vi "Lab Panel V5.31.vi"() -> ()   [LabVIEW 2017] (continued)
              tunnel: w5237 -> [w5242 _]
              tunnel: w5226 -> [_ w5275]
              tunnel: w5236 -> [_ w5274]
              tunnel: w5235 -> [_ w5273]
              tunnel: w5234 -> [_ w5272]
              tunnel: w5233 -> [_ w5271]
              tunnel: w5232 -> [_ w5270]
              tunnel: w5231 -> [_ w5269]
              tunnel: w5230 -> [_ w5268]
              tunnel: w5229 -> [_ w5267]
              tunnel: w5228 -> [_ w5266]
              tunnel: w5227 -> [_ w5265]
              tunnel: "TO (string):" -> [w5241 _]
              frame #0 {
                # "mail test"
                n2904 = case shown="True" w5242 {
                  tunnel: w5245 -> [_ w5249]
                  tunnel: w5241 -> [_ w5248]
                  tunnel: w5244 -> [_ w5247]
                  tunnel: w5243 -> [_ w5246]
                  frame False {
                  }
                  frame True {
                    n2905 = stacked-sequence {
                      seq-local: [_ _ w5259 _] -> [_ _ _ w5260]
                      tunnel: w5249 -> [w5252 _ _ w5264]
                      tunnel: w5248 -> [_ _ w5257 _]
                      tunnel: w5247 -> [_ _ w5255 _]
                      tunnel: w5246 -> [_ _ w5256 _]
                      frame #0 {
                        n2906 = Bundle(cluster=w5252, "TEST MAIL STATUS"="TEST START") -> (w5250:T8)  [unwired: 6 in]
                        n2907 = local write "MAIL SETTINGS"(w5250) -> ()
                      }
                      frame #1 {
                        n2908 = Wait (ms)(milliseconds to wait=500) -> ()  [unwired: 1 out]
                      }
                      frame #2 {
                        n2909 = call "sub vi - send mail v5.vi"("TO:"=w5257, "subject"="MAIL TEST FROM LAB PANEL", "from"=w5256, "out going server"=w5255, "message"="TEST MESSAGE") -> ("error out"=w5259:errorcluster)  [unwired: 10 in]
                      }
                      frame #3 {
                        n2910 = Bundle(cluster=w5264, "TEST MAIL"=FALSE, "TEST MAIL STATUS"="TEST END", "mail error"=w5260) -> (w5262:T8)  [unwired: 4 in]
                        n2911 = local write "MAIL SETTINGS"(w5262) -> ()
                      }
                    }
                  }
                }
              }
              frame #1 {
                # "mail report"
                n2912 = stacked-sequence {
                  seq-local: [_ w5322 _ _] -> [_ _ _ w5512]
                  seq-local: [_ _ w5425 _] -> [_ _ _ w5502]
                  seq-local: [w5289 _ _ _] -> [_ w5339 _ _]
                  seq-local: [w5288 _ _ _] -> [_ w5338 _ _]
                  seq-local: [w5286 _ _ _] -> [_ w5336 _ _]
                  seq-local: [w5287 _ _ _] -> [_ w5337 _ _]
                  seq-local: [w5285 _ _ _] -> [_ w5335 _ _]
                  seq-local: [w5284 _ _ _] -> [_ w5330 _ _]
                  seq-local: [w5283 _ _ _] -> [_ w5331 _ _]
                  seq-local: [w5282 _ _ _] -> [_ w5332 _ _]
                  seq-local: [w5281 _ _ _] -> [_ w5333 _ _]
                  seq-local: [w5280 _ _ _] -> [_ w5334 _ _]
                  tunnel: w5279 -> [_ _ _ w5513]
                  tunnel: w5278 -> [_ _ _ w5496]
                  tunnel: w5277 -> [_ _ _ w5510]
                  tunnel: w5276 -> [_ _ _ w5509]
                  tunnel: w5275 -> [w5320 _ _ w5504]
                  tunnel: w5274 -> [_ _ w5455 _]
                  tunnel: w5273 -> [_ _ w5452 _]
                  tunnel: w5272 -> [_ _ w5451 _]
                  tunnel: w5271 -> [_ _ w5450 _]
                  tunnel: w5270 -> [_ _ w5449 _]
                  tunnel: w5269 -> [_ _ w5448 _]
                  tunnel: w5268 -> [_ _ w5447 _]
                  tunnel: w5267 -> [_ _ w5446 _]
                  tunnel: w5266 -> [_ _ w5445 _]
                  tunnel: w5265 -> [_ _ w5444 _]
                  frame #0 {
                    n2913 = case shown="False" w5320 {
                      frame False {
                        n2914 = local write "mail control"("") -> ()
                      }
                      frame True {
                      }
                    }
                    n2915 = local read "SET LAB01-1"() -> (w5319:T6)
                    n2916 = local read "SET LAB01-2"() -> (w5318:T5)
                    n2917 = local read "SET LAB02-1"() -> (w5317:T5)
                    n2918 = local read "SET LAB02-2"() -> (w5316:T5)
                    n2919 = local read "SET LAB03-1"() -> (w5315:T5)
                    n2920 = local read "SET LAB04-1"() -> (w5313:T5)
                    n2921 = local read "SET LAB05-1"() -> (w5311:T5)
                    n2922 = local read "SET LAB03-2"() -> (w5314:T5)
                    n2923 = local read "SET LAB04-2"() -> (w5312:T5)
                    n2924 = local read "SET LAB05-2"() -> (w5310:T5)
                    n2925 = Unbundle(w5315) -> ("DESCRIPTION"=w5295:string)  [unwired: 4 out]
                    n2926 = Unbundle(w5314) -> ("DESCRIPTION"=w5294:string)  [unwired: 4 out]
                    n2927 = Unbundle(w5313) -> ("DESCRIPTION"=w5293:string)  [unwired: 4 out]
                    n2928 = Unbundle(w5310) -> ("DESCRIPTION"=w5290:string)  [unwired: 4 out]
                    n2929 = Unbundle(w5316) -> ("DESCRIPTION"=w5296:string)  [unwired: 4 out]
                    n2930 = Unbundle(w5312) -> ("DESCRIPTION"=w5292:string)  [unwired: 4 out]
                    n2931 = Unbundle(w5319) -> ("DESCRIPTION"=w5308:string)  [unwired: 4 out]
                    n2932 = Unbundle(w5317) -> ("DESCRIPTION"=w5297:string)  [unwired: 4 out]
                    n2933 = Unbundle(w5311) -> ("DESCRIPTION"=w5291:string)  [unwired: 4 out]
                    n2934 = Unbundle(w5318) -> ("DESCRIPTION"=w5298:string)  [unwired: 4 out]
                    n2935 = Concatenate Strings("[LAB05-2/", w5290) -> (w5280:string)
                    n2936 = Concatenate Strings("[LAB05-1/", w5291) -> (w5281:string)
                    n2937 = Concatenate Strings("[LAB04-2/", w5292) -> (w5282:string)
                    n2938 = Concatenate Strings("[LAB03-2/", w5294) -> (w5284:string)
                    n2939 = Concatenate Strings("[LAB04-1/", w5293) -> (w5283:string)
                    n2940 = Concatenate Strings("[LAB03-1/", w5295) -> (w5285:string)
                    n2941 = Concatenate Strings("[LAB01-2/", w5298) -> (w5288:string)
                    n2942 = Concatenate Strings("[LAB02-2/", w5296) -> (w5286:string)
                    n2943 = Concatenate Strings("[LAB01-1/", w5308) -> (w5289:string)
                    n2944 = Concatenate Strings("[LAB02-1/", w5297) -> (w5287:string)
                  }
                  frame #1 {
                    w5343 = "/"
                    w5344 = 2.0
                    n2945 = local read "DISP LAB01-1"() -> (w5424:T4)
                    n2946 = local read "DISP LAB01-2"() -> (w5423:T4)
                    n2947 = local read "DISP LAB02-1"() -> (w5422:T4)
                    n2948 = local read "DISP LAB03-2"() -> (w5419:T4)
                    n2949 = local read "DISP LAB02-2"() -> (w5421:T4)
                    n2950 = local read "DISP LAB03-1"() -> (w5420:T4)
                    n2951 = local read "DISP LAB04-2"() -> (w5417:T4)
                    n2952 = local read "DISP LAB04-1"() -> (w5418:T4)
                    n2953 = local read "DISP LAB05-1"() -> (w5416:T4)
                    n2954 = local read "DISP LAB05-2"() -> (w5415:T4)
                    n2955 = Unbundle By Name(w5424) -> ("CYCLE"=w5412:dbl, "MINS"=w5411:dbl, "STATUS"=w5408:string)
                    n2956 = Unbundle(w5423) -> ("CYCLE"=w5407:dbl, "MINS"=w5406:dbl, "STATUS"=w5403:string)
                    n2957 = Unbundle(w5422) -> ("CYCLE"=w5400:dbl, "MINS"=w5399:dbl, "STATUS"=w5398:string)
                    n2958 = Unbundle(w5419) -> ("CYCLE"=w5387:dbl, "MINS"=w5386:dbl, "STATUS"=w5383:string)
                    n2959 = Unbundle(w5420) -> ("CYCLE"=w5392:dbl, "MINS"=w5391:dbl, "STATUS"=w5388:string)
                    n2960 = Unbundle(w5421) -> ("CYCLE"=w5397:dbl, "MINS"=w5396:dbl, "STATUS"=w5393:string)
                    n2961 = Unbundle(w5418) -> ("CYCLE"=w5382:dbl, "MINS"=w5381:dbl, "STATUS"=w5378:string)
                    n2962 = Unbundle(w5417) -> ("CYCLE"=w5377:dbl, "MINS"=w5376:dbl, "STATUS"=w5373:string)
                    n2963 = Unbundle(w5416) -> ("CYCLE"=w5372:dbl, "MINS"=w5371:dbl, "STATUS"=w5368:string)
                    n2964 = Unbundle(w5415) -> ("CYCLE"=w5414:dbl, "MINS"=w5413:dbl, "STATUS"=w5365:string)
                    n2965 = Number To Decimal String(number=w5400) -> (decimal integer string=w5402:string)  [unwired: 1 in]
                    n2966 = Number To Decimal String(number=w5397) -> (decimal integer string=w5395:string)  [unwired: 1 in]
                    n2967 = Number To Decimal String(number=w5392) -> (decimal integer string=w5390:string)  [unwired: 1 in]
                    n2968 = Number To Decimal String(number=w5407) -> (decimal integer string=w5405:string)  [unwired: 1 in]
                    n2969 = Number To Decimal String(number=w5387) -> (decimal integer string=w5385:string)  [unwired: 1 in]
                    n2970 = Number To Decimal String(number=w5412) -> (decimal integer string=w5410:string)  [unwired: 1 in]
                    n2971 = Number To Decimal String(number=w5414) -> (decimal integer string=w5367:string)  [unwired: 1 in]
                    n2972 = Number To Decimal String(number=w5382) -> (decimal integer string=w5380:string)  [unwired: 1 in]
                    n2973 = Number To Decimal String(number=w5377) -> (decimal integer string=w5375:string)  [unwired: 1 in]
                    n2974 = Number To Decimal String(number=w5372) -> (decimal integer string=w5370:string)  [unwired: 1 in]
                    n2975 = Number To Fractional String(number=w5399, precision (6)=w5344) -> (F-format string=w5401:string)  [unwired: 2 in]
                    n2976 = Number To Fractional String(number=w5386, precision (6)=w5344) -> (F-format string=w5384:string)  [unwired: 2 in]
                    n2977 = Number To Fractional String(number=w5396, precision (6)=w5344) -> (F-format string=w5394:string)  [unwired: 2 in]
                    n2978 = Number To Fractional String(number=w5391, precision (6)=w5344) -> (F-format string=w5389:string)  [unwired: 2 in]
                    n2979 = Number To Fractional String(number=w5376, precision (6)=w5344) -> (F-format string=w5374:string)  [unwired: 2 in]
                    n2980 = Number To Fractional String(number=w5381, precision (6)=w5344) -> (F-format string=w5379:string)  [unwired: 2 in]
                    n2981 = Number To Fractional String(number=w5406, precision (6)=w5344) -> (F-format string=w5404:string)  [unwired: 2 in]
                    n2982 = Number To Fractional String(number=w5371, precision (6)=w5344) -> (F-format string=w5369:string)  [unwired: 2 in]
                    n2983 = Number To Fractional String(number=w5411, precision (6)=w5344) -> (F-format string=w5409:string)  [unwired: 2 in]
                    n2984 = Number To Fractional String(number=w5413, precision (6)=w5344) -> (F-format string=w5366:string)  [unwired: 2 in]
                    n2985 = Concatenate Strings(w5343, w5385, w5343, w5384, w5343, w5383) -> (w5359:string)
                    n2986 = Concatenate Strings(w5343, w5380, w5343, w5379, w5343, w5378) -> (w5358:string)
                    n2987 = Concatenate Strings(w5343, w5375, w5343, w5374, w5343, w5373) -> (w5357:string)
                    n2988 = Concatenate Strings(w5343, w5370, w5343, w5369, w5343, w5368) -> (w5356:string)
                    n2989 = Concatenate Strings(w5343, w5367, w5343, w5366, w5343, w5365) -> (w5355:string)
                    n2990 = Concatenate Strings(w5343, w5410, w5343, w5409, w5343, w5408) -> (w5364:string)
                    n2991 = Concatenate Strings(w5343, w5390, w5343, w5389, w5343, w5388) -> (w5360:string)
                    n2992 = Concatenate Strings(w5343, w5405, w5343, w5404, w5343, w5403) -> (w5363:string)
                    n2993 = Concatenate Strings(w5343, w5402, w5343, w5401, w5343, w5398) -> (w5362:string)
                    n2994 = Concatenate Strings(w5343, w5395, w5343, w5394, w5343, w5393) -> (w5361:string)
                    n2995 = Concatenate Strings("]", "\r") -> (w5340:string)
                    n2996 = Concatenate Strings(w5335, w5360, w5340) -> (w5350:string)
                    n2997 = Concatenate Strings(w5337, w5362, w5340) -> (w5352:string)
                    n2998 = Concatenate Strings(w5336, w5361, w5340) -> (w5351:string)
                    n2999 = Concatenate Strings(w5332, w5357, w5340) -> (w5347:string)
                    n3000 = Concatenate Strings(w5333, w5356, w5340) -> (w5348:string)
                    n3001 = Concatenate Strings(w5331, w5358, w5340) -> (w5346:string)
                    n3002 = Concatenate Strings(w5330, w5359, w5340) -> (w5345:string)
                    n3003 = Concatenate Strings(w5334, w5355, w5340) -> (w5349:string)
                    n3004 = Concatenate Strings(w5338, w5363, w5340) -> (w5353:string)
                    n3005 = Concatenate Strings(w5339, w5364, w5340) -> (w5354:string)
                    n3006 = Concatenate Strings(w5354, w5353, w5352, w5351, w5350, w5345, w5346, w5347, w5348, w5349) -> (w5323:string)
                    n3007 = Concatenate Strings("[PANEL/", "DESC/", "CYCLES/", "MINS/", "STATUS]", "\r", w5323) -> (w5322:string)
                    "MAIL REPORT" <- w5322
                    n3008 = global write "Global display 3.vi" "log all"(w5322) -> ()
                  }
                  frame #2 {
                    w5453 = "END"
                    n3009 = local read "mail control"() -> (w5454:string)
                    n3010 = case shown="False" w5449 {
                      tunnel: w5454 -> [w5478 _]
                      tunnel: w5453 -> [w5477 _]
                      tunnel: [w5476 FALSE] -> w5439
                      frame False {
                        n3011 = Equal?(x=w5478, y=w5477) -> (x = y?=w5476:bool)
                      }
                      frame True {
                      }
                    }
                    n3012 = case shown="False" w5455 {
                      tunnel: w5454 -> [w5494 _]
                      tunnel: w5453 -> [w5493 _]
                      tunnel: [w5492 FALSE] -> w5443
                      frame False {
                        n3013 = Equal?(x=w5494, y=w5493) -> (x = y?=w5492:bool)
                      }
                      frame True {
                      }
                    }
                    n3014 = case shown="False" w5452 {
                      tunnel: w5454 -> [w5490 _]
                      tunnel: w5453 -> [w5489 _]
                      tunnel: [w5488 FALSE] -> w5442
                      frame False {
                        n3015 = Equal?(x=w5490, y=w5489) -> (x = y?=w5488:bool)
                      }
                      frame True {
                      }
                    }
                    n3016 = case shown="False" w5450 {
                      tunnel: w5454 -> [w5482 _]
                      tunnel: w5453 -> [w5481 _]
                      tunnel: [w5480 FALSE] -> w5440
                      frame False {
                        n3017 = Equal?(x=w5482, y=w5481) -> (x = y?=w5480:bool)
                      }
                      frame True {
                      }
                    }
                    n3018 = case shown="False" w5451 {
                      tunnel: w5454 -> [w5486 _]
                      tunnel: w5453 -> [w5485 _]
                      tunnel: [w5484 FALSE] -> w5441
                      frame False {
                        n3019 = Equal?(x=w5486, y=w5485) -> (x = y?=w5484:bool)
                      }
                      frame True {
                      }
                    }
                    n3020 = Or(x=w5441, y=w5440) -> (x .or. y?=w5432:bool)
                    n3021 = Or(x=w5443, y=w5442) -> (x .or. y?=w5433:bool)
                    n3022 = Or(x=w5433, y=w5432) -> (x .or. y?=w5428:bool)
                    n3023 = case shown="False" w5445 {
                      tunnel: w5454 -> [w5462 _]
                      tunnel: w5453 -> [w5461 _]
                      tunnel: [w5460 FALSE] -> w5434
                      frame False {
                        n3024 = Equal?(x=w5462, y=w5461) -> (x = y?=w5460:bool)
                      }
                      frame True {
                      }
                    }
                    n3025 = case shown="False" w5444 {
                      tunnel: w5454 -> [w5458 _]
                      tunnel: w5453 -> [w5457 _]
                      tunnel: [w5456 FALSE] -> w5438
                      frame False {
                        n3026 = Equal?(x=w5458, y=w5457) -> (x = y?=w5456:bool)
                      }
                      frame True {
                      }
                    }
                    n3027 = case shown="False" w5446 {
                      tunnel: w5454 -> [w5466 _]
                      tunnel: w5453 -> [w5465 _]
                      tunnel: [w5464 FALSE] -> w5435
                      frame False {
                        n3028 = Equal?(x=w5466, y=w5465) -> (x = y?=w5464:bool)
                      }
                      frame True {
                      }
                    }
                    n3029 = case shown="False" w5448 {
                      tunnel: w5454 -> [w5474 _]
                      tunnel: w5453 -> [w5473 _]
                      tunnel: [w5472 FALSE] -> w5437
                      frame False {
                        n3030 = Equal?(x=w5474, y=w5473) -> (x = y?=w5472:bool)
                      }
                      frame True {
                      }
                    }
                    n3031 = case shown="False" w5447 {
                      tunnel: w5454 -> [w5470 _]
                      tunnel: w5453 -> [w5469 _]
                      tunnel: [w5468 FALSE] -> w5436
                      frame False {
                        n3032 = Equal?(x=w5470, y=w5469) -> (x = y?=w5468:bool)
                      }
                      frame True {
                      }
                    }
                    n3033 = Or(x=w5437, y=w5436) -> (x .or. y?=w5431:bool)
                    n3034 = Or(x=w5435, y=w5434) -> (x .or. y?=w5430:bool)
                    n3035 = Or(x=w5438, y=w5439) -> (x .or. y?=w5426:bool)
                    n3036 = Or(x=w5431, y=w5430) -> (x .or. y?=w5429:bool)
                    n3037 = Or(x=w5428, y=w5429) -> (x .or. y?=w5427:bool)
                    n3038 = Or(x=w5427, y=w5426) -> (x .or. y?=w5425:bool)
                  }
                  frame #3 {
                    n3039 = local read "on loops"() -> (w5508:dbl)
                    n3040 = local read "jig cycle"() -> (w5505:dbl)
                    n3041 = local read "Send Mail Now"() -> (w5499:bool)
                    n3042 = Add(x=w5508, y=5.0) -> (x+y=w5506:dbl)
                    n3043 = Equal?(x=w5505, y=w5506) -> (x = y?=w5500:bool)
                    n3044 = And(x=w5500, y=w5499) -> (x .and. y?=w5498:bool)
                    n3045 = And(x=w5504, y=w5500) -> (x .and. y?=w5503:bool)
                    n3046 = And(x=w5503, y=w5502) -> (x .and. y?=w5501:bool)
                    n3047 = Or(x=w5501, y=w5498) -> (x .or. y?=w5497:bool)
                    n3048 = case shown="True" w5497 {
                      tunnel: w5513 -> [_ w5519]
                      tunnel: w5512 -> [_ w5518]
                      tunnel: "Lab Panel Test Status" -> [_ w5517]
                      tunnel: w5510 -> [_ w5516]
                      tunnel: w5509 -> [_ w5515]
                      tunnel: w5496 -> [_ w5514]
                      frame False {
                      }
                      frame True {
                        n3049 = stacked-sequence {
                          tunnel: w5519 -> [w5528 _]
                          tunnel: w5518 -> [w5527 _]
                          tunnel: w5517 -> [w5526 _]
                          tunnel: w5516 -> [w5525 _]
                          tunnel: w5515 -> [w5524 _]
                          tunnel: w5514 -> [w5523 _]
                          frame #0 {
                            n3050 = call "sub vi - send mail v5.vi"("TO:"=w5528, "subject"=w5526, "Info"="Test station status report", "from"=w5524, "out going server"=w5525, "message"=w5527) -> ("error out"=w5522:errorcluster)  [unwired: 9 in]
                            n3051 = Bundle(cluster=w5523, "mail error"=w5522) -> (w5521:T8)  [unwired: 6 in]
                            n3052 = local write "MAIL SETTINGS"(w5521) -> ()
                          }
                          frame #1 {
                            n3053 = local write "mail control"("") -> ()
                            n3054 = local write "Send Mail Now"(FALSE) -> ()
                          }
                        }
                      }
                    }
                  }
                }
              }
            }
          }
          frame #20 {
            # "save jig cycle values once all run switches are off"
            n3055 = stacked-sequence {
              tunnel: w5540 -> [_ w5569]
              tunnel: w5539 -> [_ w5568]
              tunnel: w5538 -> [_ w5567]
              tunnel: w5537 -> [_ w5566]
              tunnel: w5536 -> [_ w5565]
              tunnel: w5535 -> [_ w5564]
              tunnel: w5534 -> [_ w5563]
              tunnel: w5533 -> [_ w5562]
              tunnel: w5532 -> [_ w5561]
              tunnel: w5531 -> [_ w5560]
              frame #0 {
              }
              frame #1 {
                n3056 = Not(x=w5560) -> (.not. x?=w5543:bool)
                n3057 = Not(x=w5568) -> (.not. x?=w5558:bool)
                n3058 = Not(x=w5565) -> (.not. x?=w5553:bool)
                n3059 = Not(x=w5563) -> (.not. x?=w5549:bool)
                n3060 = Not(x=w5561) -> (.not. x?=w5545:bool)
                n3061 = Not(x=w5569) -> (.not. x?=w5559:bool)
                n3062 = Not(x=w5567) -> (.not. x?=w5557:bool)
                n3063 = Not(x=w5564) -> (.not. x?=w5551:bool)
                n3064 = Not(x=w5566) -> (.not. x?=w5555:bool)
                n3065 = Not(x=w5562) -> (.not. x?=w5547:bool)
                n3066 = local read "Save JC"() -> (w5571:bool)
                n3067 = And(x=w5559, y=w5558) -> (x .and. y?=w5556:bool)
                n3068 = And(x=w5556, y=w5557) -> (x .and. y?=w5554:bool)
                n3069 = And(x=w5554, y=w5555) -> (x .and. y?=w5552:bool)
                n3070 = And(x=w5552, y=w5553) -> (x .and. y?=w5550:bool)
                n3071 = And(x=w5550, y=w5551) -> (x .and. y?=w5548:bool)
                n3072 = And(x=w5548, y=w5549) -> (x .and. y?=w5546:bool)
                n3073 = And(x=w5546, y=w5547) -> (x .and. y?=w5544:bool)
                n3074 = And(x=w5544, y=w5545) -> (x .and. y?=w5542:bool)
                n3075 = And(x=w5542, y=w5543) -> (x .and. y?=w5541:bool)
                n3076 = And(x=w5541, y=w5571) -> (x .and. y?=w5570:bool)
                n3077 = case shown="True" w5570 {
                  tunnel: w5541 -> [w5572 _]
                  frame False {
                    n3078 = case shown="False" w5572 {
                      frame False {
                        n3079 = local write "Save JC"(TRUE) -> ()
                      }
                      frame True {
                      }
                    }
                  }
                  frame True {
                    n3080 = stacked-sequence {
                      frame #0 {
                        n3081 = String To Path(string="c:\\crabtree\\Jig Cycles\\") -> (path=w5584:path)
                        n3082 = Build Path(base path=w5584, name or relative path="jigcycles.bin") -> (appended path=w5582:path)
                        n3083 = Create Folder(path (use dialog)=w5584) -> (error out=w5586:errorcluster)  [unwired: 2 in, 2 out]
                        n3084 = local read "JIG RELAY CYCLES"() -> (w5576:T9)
                        n3085 = call <vilib>:"Clear Errors.vi"("error in (no error)"=w5586) -> ()  [unwired: 5 in, 2 out]
                        n3086 = local write "Save JC"(FALSE) -> ()
                        n3087 = Open/Create/Replace File(file path (use dialog)=w5582, operation (0:open)=T18."replace or create") -> (refnum out=w5580:refnum<file>, error out=w5581:errorcluster)  [unwired: 4 in, 1 out]
                        n3088 = Write to Binary File(file (use dialog)=w5580, data=w5576, error in=w5581) -> (refnum out=w5579:refnum<file>, error out=w5578:errorcluster)  [unwired: 3 in, 1 out]
                        n3089 = Close File(refnum=w5579, error in=w5578) -> (error out=w5577:errorcluster)  [unwired: 1 out]
                        n3090 = local write "data file error"(w5577) -> ()
                      }
                      frame #1 {
                        n3091 = local read "JIG RELAY CYCLES"() -> (w5609:T9)
                        n3092 = Unbundle By Name(w5609) -> ("LAB01-1"=w5604:dbl, "LAB01-2"=w5603:dbl, "LAB02-1"=w5601:dbl, "LAB02-2"=w5600:dbl, "LAB03-1"=w5598:dbl, "LAB03-2"=w5595:dbl, "LAB04-1"=w5594:dbl, "LAB04-2"=w5592:dbl, "LAB05-1"=w5590:dbl, "LAB05-2"=w5588:dbl)
                        n3093 = stacked-sequence {
                          tunnel: w5604 -> [w5612 _ _ _ _ _ _ _ _ _]
                          tunnel: 1000000 -> [w5615 w5625 w5635 w5645 w5655 w5665 w5675 w5685 w5695 w5705]
                          tunnel: [w5613 _ _ _ _ _ _ _ _ _] -> w5607
                          tunnel: "TEST STATION HAS REACHED 1 MILLION CYCLES, REPLACE  CONTROL RELAYS" -> [w5611 w5623 w5633 w5643 w5653 w5663 w5673 w5683 w5693 w5703]
                          tunnel: [_ w5622 _ _ _ _ _ _ _ _] -> w5605
                          tunnel: w5603 -> [_ w5621 _ _ _ _ _ _ _ _]
                          tunnel: [_ _ w5632 _ _ _ _ _ _ _] -> w5602
                          tunnel: w5601 -> [_ _ w5631 _ _ _ _ _ _ _]
                          tunnel: w5600 -> [_ _ _ w5642 _ _ _ _ _ _]
                          tunnel: [_ _ _ w5641 _ _ _ _ _ _] -> w5599
                          tunnel: w5598 -> [_ _ _ _ w5652 _ _ _ _ _]
                          tunnel: [_ _ _ _ w5651 _ _ _ _ _] -> w5597
                          tunnel: [_ _ _ _ _ w5662 _ _ _ _] -> w5596
                          tunnel: w5595 -> [_ _ _ _ _ w5661 _ _ _ _]
                          tunnel: w5594 -> [_ _ _ _ _ _ w5672 _ _ _]
                          tunnel: [_ _ _ _ _ _ w5671 _ _ _] -> w5593
                          tunnel: w5592 -> [_ _ _ _ _ _ _ w5682 _ _]
                          tunnel: [_ _ _ _ _ _ _ w5681 _ _] -> w5591
                          tunnel: w5590 -> [_ _ _ _ _ _ _ _ w5692 _]
                          tunnel: [_ _ _ _ _ _ _ _ w5691 _] -> w5589
                          tunnel: w5588 -> [_ _ _ _ _ _ _ _ _ w5702]
                          tunnel: [_ _ _ _ _ _ _ _ _ w5701] -> w5587
                          frame #0 {
                            n3094 = Greater?(x=w5612, y=w5615) -> (0:w5614:bool)
                            n3095 = case shown="True" w5614 {
                              tunnel: [w5616 0] -> w5613
                              tunnel: w5612 -> [w5616 _]
                              tunnel: w5611 -> [_ w5617]
                              frame False {
                              }
                              frame True {
                                n3096 = Concatenate Strings("LA01-1 ", w5617) -> (w5620:string)
                                n3097 = One Button Dialog(message=w5620) -> ()  [unwired: 1 in, 1 out]
                              }
                            }
                          }
                          frame #1 {
                            n3098 = Greater?(x=w5621, y=w5625) -> (0:w5624:bool)
                            n3099 = case shown="True" w5624 {
                              tunnel: [w5626 0] -> w5622
                              tunnel: w5621 -> [w5626 _]
                              tunnel: w5623 -> [_ w5627]
                              frame False {
                              }
                              frame True {
                                n3100 = Concatenate Strings("LA01-2 ", w5627) -> (w5630:string)
                                n3101 = One Button Dialog(message=w5630) -> ()  [unwired: 1 in, 1 out]
                              }
                            }
                          }
                          frame #2 {
                            n3102 = Greater?(x=w5631, y=w5635) -> (0:w5634:bool)
                            n3103 = case shown="True" w5634 {
                              tunnel: [w5636 0] -> w5632
                              tunnel: w5631 -> [w5636 _]
                              tunnel: w5633 -> [_ w5637]
                              frame False {
                              }
                              frame True {
                                n3104 = Concatenate Strings("LA02-1 ", w5637) -> (w5640:string)
                                n3105 = One Button Dialog(message=w5640) -> ()  [unwired: 1 in, 1 out]
                              }
                            }
                          }
                          frame #3 {
                            n3106 = Greater?(x=w5642, y=w5645) -> (0:w5644:bool)
                            n3107 = case shown="True" w5644 {
                              tunnel: [w5646 0] -> w5641
                              tunnel: w5642 -> [w5646 _]
                              tunnel: w5643 -> [_ w5647]
                              frame False {
                              }
                              frame True {
                                n3108 = Concatenate Strings("LA02-2 ", w5647) -> (w5650:string)
                                n3109 = One Button Dialog(message=w5650) -> ()  [unwired: 1 in, 1 out]
                              }
                            }
                          }
                          frame #4 {
                            n3110 = Greater?(x=w5652, y=w5655) -> (0:w5654:bool)
                            n3111 = case shown="True" w5654 {
                              tunnel: [w5656 0] -> w5651
                              tunnel: w5652 -> [w5656 _]
                              tunnel: w5653 -> [_ w5657]
                              frame False {
                              }
                              frame True {
                                n3112 = Concatenate Strings("LA03-1 ", w5657) -> (w5660:string)
                                n3113 = One Button Dialog(message=w5660) -> ()  [unwired: 1 in, 1 out]
                              }
                            }
                          }
                          frame #5 {
                            n3114 = Greater?(x=w5661, y=w5665) -> (0:w5664:bool)
                            n3115 = case shown="True" w5664 {
                              tunnel: [w5666 0] -> w5662
                              tunnel: w5661 -> [w5666 _]
                              tunnel: w5663 -> [_ w5667]
                              frame False {
                              }
                              frame True {
                                n3116 = Concatenate Strings("LA03-2 ", w5667) -> (w5670:string)
                                n3117 = One Button Dialog(message=w5670) -> ()  [unwired: 1 in, 1 out]
                              }
                            }
                          }
                          frame #6 {
                            n3118 = Greater?(x=w5672, y=w5675) -> (0:w5674:bool)
                            n3119 = case shown="True" w5674 {
                              tunnel: [w5676 0] -> w5671
                              tunnel: w5672 -> [w5676 _]
                              tunnel: w5673 -> [_ w5677]
                              frame False {
                              }
                              frame True {
                                n3120 = Concatenate Strings("LA04-1 ", w5677) -> (w5680:string)
                                n3121 = One Button Dialog(message=w5680) -> ()  [unwired: 1 in, 1 out]
                              }
                            }
                          }
                          frame #7 {
                            n3122 = Greater?(x=w5682, y=w5685) -> (0:w5684:bool)
                            n3123 = case shown="True" w5684 {
                              tunnel: [w5686 0] -> w5681
                              tunnel: w5682 -> [w5686 _]
                              tunnel: w5683 -> [_ w5687]
                              frame False {
                              }
                              frame True {
                                n3124 = Concatenate Strings("LA04-2 ", w5687) -> (w5690:string)
                                n3125 = One Button Dialog(message=w5690) -> ()  [unwired: 1 in, 1 out]
                              }
                            }
                          }
                          frame #8 {
                            n3126 = Greater?(x=w5692, y=w5695) -> (0:w5694:bool)
                            n3127 = case shown="True" w5694 {
                              tunnel: [w5696 0] -> w5691
                              tunnel: w5692 -> [w5696 _]
                              tunnel: w5693 -> [_ w5697]
                              frame False {
                              }
                              frame True {
                                n3128 = Concatenate Strings("LA05-1 ", w5697) -> (w5700:string)
                                n3129 = One Button Dialog(message=w5700) -> ()  [unwired: 1 in, 1 out]
                              }
                            }
                          }
                          frame #9 {
                            n3130 = Greater?(x=w5702, y=w5705) -> (0:w5704:bool)
                            n3131 = case shown="True" w5704 {
                              tunnel: [w5706 0] -> w5701
                              tunnel: w5702 -> [w5706 _]
                              tunnel: w5703 -> [_ w5707]
                              frame False {
                              }
                              frame True {
                                n3132 = Concatenate Strings("LA05-2 ", w5707) -> (w5710:string)
                                n3133 = One Button Dialog(message=w5710) -> ()  [unwired: 1 in, 1 out]
                              }
                            }
                          }
                        }
                        n3134 = Bundle By Name(cluster=w5609, "LAB01-1"=w5607, "LAB01-2"=w5605, "LAB02-1"=w5602, "LAB02-2"=w5599, "LAB03-1"=w5597, "LAB03-2"=w5596, "LAB04-1"=w5593, "LAB04-2"=w5591, "LAB05-1"=w5589, "LAB05-2"=w5587) -> (w5608:T9)
                        n3135 = local write "JIG RELAY CYCLES"(w5608) -> ()
                      }
                    }
                  }
                }
              }
            }
          }
          frame #21 {
            # "get temperature values"
            n3136 = local read "Simulate"() -> (w5723:bool)
            n3137 = local read "Temp Test Cal"() -> (w5720:dbl)
            n3138 = stacked-sequence {
              seq-local: [_ w5730 _] -> [_ _ w5775]
              tunnel: w5723 -> [_ _ w5788]
              tunnel: T15 {"1  (A) cal"=1.0, "1 (V) cal"=1.0, "1 (PF) cal"=1.0, "1 (TL) cal"=1.0, "1 (TN) cal"=1.0, "2 (A) cal"=1.0, "2 (V) cal"=1.0, "2 (PF) cal"=1.0, "2 (TL) cal"=1.0, "2 (TN) cal"=1.0} ("CAL LAB01") -> [_ _ w5787]
              tunnel: w5721 -> [_ _ w5786]
              tunnel: w5720 -> [_ _ w5785]
              tunnel: w5719 -> [_ _ w5784]
              tunnel: w5718 -> [_ _ w5783]
              tunnel: w5717 -> [_ _ w5782]
              tunnel: w5716 -> [_ _ w5781]
              tunnel: w5715 -> [_ _ w5780]
              tunnel: w5714 -> [_ _ w5779]
              tunnel: w5713 -> [_ _ w5778]
              tunnel: w5712 -> [_ _ w5777]
              tunnel: w5711 -> [_ _ w5776]
              frame #0 {
                n3139 = case shown="True" "Open Com Port" {
                  frame False {
                  }
                  frame True {
                    n3140 = local read "Select COM port"() -> (w5728:refnum<visa-resource-name>)
                    n3141 = call "sub vi-open serial port v1.vi"("Select COM port"=w5728) -> ("Error"=w5727:bool, "LOOPS"=w5726:i32, "VISA Com out"=w5725:refnum<visa-resource-name>)  [unwired: 12 in]
                    n3142 = local write "Com setup loops"(w5726) -> ()
                    n3143 = local write "Com Port Status"(w5727) -> ()
                    n3144 = local write "VISA Com out"(w5725) -> ()
                    n3145 = global write "Global 1.vi" "COM port"(w5725) -> ()
                  }
                }
              }
              frame #1 {
                # "only get temperature from initial valid temperature circuits, circuits detected at startup time"
                n3146 = local read "VISA Com out"() -> (w5738:refnum<visa-resource-name>)
                n3147 = global write "Global 1.vi" "COM port"(w5738) -> ()
                n3148 = local read "Temp read loop"() -> (w5735:dbl)
                n3149 = global write "Global 1.vi" "tmp dly lps"("Temp Delay Lps") -> ()
                n3150 = global write "Global 1.vi" "dly value"("Temp Value") -> ()
                n3151 = local read "jig cycle"() -> (w5739:dbl)
                n3152 = local read "on loops"() -> (w5741:dbl)
                n3153 = Equal?(x=w5735, y=1) -> (x = y?=w5732:bool)
                n3154 = Add(x=w5741, y=6) -> (x+y=w5742:dbl)
                n3155 = Equal?(x=w5739, y=w5742) -> (x = y?=w5733:bool)
                n3156 = And(x=w5733, y=w5732) -> (x .and. y?=w5731:bool)
                n3157 = Or(x=w5731, y="Read Temp") -> (x .or. y?=w5730:bool)
                n3158 = case shown="True" w5730 {
                  frame False {
                  }
                  frame True {
                    n3159 = local read "Simulate"() -> (w5744:bool)
                    n3160 = local write "TEMP"(TRUE) -> ()
                    n3161 = local write "Read Temp"(FALSE) -> ()
                    n3162 = stacked-sequence {
                      tunnel: 1.0 -> [_ _ _ _ w5774]
                      tunnel: w5744 -> [_ _ _ _ w5773]
                      frame #0 {
                        # "only switch relay on to reset temp circuits if busy testing"
                        n3163 = disable-structure shown="Disabled" {
                          frame Disabled {
                            n3164 = local read "Any Test Running"() -> ()  [unwired: 1 out]
                          }
                          frame Enabled {
                          }
                        }
                        n3165 = local read "USB OUT 0"() -> (w5748:bool[])
                        n3166 = local read "USB OUT 2"() -> (w5750:bool[])
                        n3167 = local read "USB OUT 1"() -> (w5749:bool[])
                        n3168 = Insert Into Array(array=w5750, index=7, new element=TRUE) -> (w5751:bool[])
                        n3169 = call "sub vi - Drive Relays All v6.vi"("Array #2"=w5751, "Array #1"=w5749, "Array #0"=w5748) -> ()  [unwired: 8 in, 1 out]
                      }
                      frame #1 {
                        # "time delay"
                        n3170 = Wait (ms)(milliseconds to wait=500) -> ()  [unwired: 1 out]
                      }
                      frame #2 {
                        # "switch relay off"
                        n3171 = local read "USB OUT 0"() -> (w5754:bool[])
                        n3172 = local read "USB OUT 2"() -> (w5756:bool[])
                        n3173 = local read "USB OUT 1"() -> (w5755:bool[])
                        n3174 = Insert Into Array(array=w5756, index=7, new element=FALSE) -> (w5757:bool[])
                        n3175 = call "sub vi - Drive Relays All v6.vi"("Array #2"=w5757, "Array #1"=w5755, "Array #0"=w5754) -> ()  [unwired: 8 in, 1 out]
                      }
                      frame #3 {
                        # "time delay"
                        n3176 = Wait (ms)(milliseconds to wait=300) -> ()  [unwired: 1 out]
                      }
                      frame #4 {
                        # "read all valid temp circuits"
                        n3177 = local read "LAB01-TP"() -> (w5766:bool)
                        n3178 = local read "LAB03-TP"() -> (w5764:bool)
                        n3179 = local read "LAB02-TP"() -> (w5765:bool)
                        n3180 = local read "LAB04-TP"() -> (w5763:bool)
                        n3181 = local read "LAB05-TP"() -> (w5767:bool)
                        n3182 = call "sub vi - GET ALL TEMP v7.vi"("LA01-EN"=w5766, "simulate"=w5773, "LA02-EN"=w5765, "LA03-EN"=w5764, "LA04-EN"=w5763, "LA05-EN"=w5767, "Gen Cal Value"=w5774) -> ("LOOP TIME"=→"Read Time":dbl, "LA01 TEMP"=w5772:T27, "LA02 TEMP"=w5771:T27, "LA03 TEMP"=w5770:T27, "LA04 TEMP"=w5769:T27, "error"=→"Error Temp":bool, "LA05 TEMP"=w5768:T27)  [unwired: 1 in, 1 out]
                        n3183 = local write "LAB01 TEMP"(w5772) -> ()
                        n3184 = local write "LAB02 TEMP"(w5771) -> ()
                        n3185 = local write "LAB03 TEMP"(w5770) -> ()
                        n3186 = local write "LAB04 TEMP"(w5769) -> ()
                        n3187 = local write "LAB05 TEMP"(w5768) -> ()
                      }
                    }
                  }
                }
              }
              frame #2 {
                n3188 = case shown="True" w5775 {
                  tunnel: w5788 -> [_ w5801]
                  tunnel: w5787 -> [_ w5800]
                  tunnel: w5786 -> [_ w5799]
                  tunnel: w5785 -> [_ w5798]
                  tunnel: w5784 -> [_ w5797]
                  tunnel: w5783 -> [_ w5796]
                  tunnel: w5782 -> [_ w5795]
                  tunnel: w5781 -> [_ w5794]
                  tunnel: w5780 -> [_ w5793]
                  tunnel: w5779 -> [_ w5792]
                  tunnel: w5778 -> [_ w5791]
                  tunnel: w5777 -> [_ w5790]
                  tunnel: w5776 -> [_ w5789]
                  frame False {
                  }
                  frame True {
                    n3189 = stacked-sequence {
                      tunnel: w5801 -> [_ w5814 w5859 w5904 w5949 w5994 _]
                      tunnel: w5800 -> [_ w5813 w5858 w5903 w5948 w5993 _]
                      tunnel: w5799 -> [_ w5803 _ _ _ _ _]
                      tunnel: w5798 -> [_ w5808 w5857 w5902 w5947 w5992 _]
                      tunnel: w5797 -> [_ w5802 _ _ _ _ _]
                      tunnel: w5796 -> [_ _ w5848 _ _ _ _]
                      tunnel: w5795 -> [_ _ w5847 _ _ _ _]
                      tunnel: w5794 -> [_ _ _ w5893 _ _ _]
                      tunnel: w5793 -> [_ _ _ w5892 _ _ _]
                      tunnel: w5792 -> [_ _ _ _ w5938 _ _]
                      tunnel: w5791 -> [_ _ _ _ w5937 _ _]
                      tunnel: w5790 -> [_ _ _ _ _ w5983 _]
                      tunnel: w5789 -> [_ _ _ _ _ w5982 _]
                      frame #0 {
                      }
                      frame #1 {
                        n3190 = case shown="False" w5814 {
                          tunnel: [w5845 w5846] -> w5830
                          tunnel: w5813 -> [_ w5846]
                          frame False {
                            n3191 = local read "CAL LAB01"() -> (w5845:T15)
                          }
                          frame True {
                          }
                        }
                        n3192 = local read "TEMP LA01"() -> (w5821:T10)
                        n3193 = local read "LAB01 TEMP"() -> (w5820:T13)
                        n3194 = call "sub vi - temperature delay v4.vi"("2-run"=w5802, "1-run"=w5803, "temp values IN"=w5821, "temp signals"=w5820) -> ("T2-N"=w5816:dbl, "T2-L"=w5817:dbl, "T1-N"=w5818:dbl, "T1-L"=w5819:dbl, "temp values OUT"=w5815:T47)  [unwired: 3 in]
                        n3195 = Unbundle By Name(w5830) -> ("1 (TL) cal"=w5825:dbl, "1 (TN) cal"=w5824:dbl, "2 (TL) cal"=w5823:dbl, "2 (TN) cal"=w5822:dbl)  [unwired: 6 out]
                        n3196 = local write "TEMP LA01"(w5815) -> ()
                        n3197 = Multiply(x=w5819, y=w5825) -> (x*y=w5812:dbl)
                        n3198 = Multiply(x=w5818, y=w5824) -> (x*y=w5810:dbl)
                        n3199 = Multiply(x=w5817, y=w5823) -> (x*y=w5807:dbl)
                        n3200 = Multiply(x=w5816, y=w5822) -> (x*y=w5806:dbl)
                        n3201 = case shown="True" w5803 {
                          tunnel: w5812 -> [w5839 w5844]
                          tunnel: w5808 -> [_ w5842]
                          tunnel: [w5839 w5843] -> w5811
                          tunnel: w5810 -> [w5838 w5841]
                          tunnel: [w5838 w5840] -> w5809
                          frame False {
                          }
                          frame True {
                            n3202 = Multiply(x=w5842, y=w5841) -> (x*y=w5840:dbl)
                            n3203 = Multiply(x=w5842, y=w5844) -> (x*y=w5843:dbl)
                          }
                        }
                        n3204 = case shown="True" w5802 {
                          tunnel: w5807 -> [w5832 w5837]
                          tunnel: w5808 -> [_ w5835]
                          tunnel: [w5832 w5836] -> w5805
                          tunnel: w5806 -> [w5831 w5834]
                          tunnel: [w5831 w5833] -> w5804
                          frame False {
                          }
                          frame True {
                            n3205 = Multiply(x=w5835, y=w5834) -> (x*y=w5833:dbl)
                            n3206 = Multiply(x=w5835, y=w5837) -> (x*y=w5836:dbl)
                          }
                        }
                        n3207 = local read "SIG LAB01-2"() -> (w5827:T2)
                        n3208 = local read "SIG LAB01-1"() -> (w5829:T2)
                        n3209 = Bundle By Name(cluster=w5829, "Tmp Live"=w5811, "Tmp Neut"=w5809) -> (w5828:T2)
                        n3210 = Bundle By Name(cluster=w5827, "Tmp Live"=w5805, "Tmp Neut"=w5804) -> (w5826:T2)
                        n3211 = local write "SIG LAB01-1"(w5828) -> ()
                        n3212 = local write "SIG LAB01-2"(w5826) -> ()
                      }
                      frame #2 {
                        n3213 = case shown="True" w5859 {
                          tunnel: [w5890 w5891] -> w5875
                          tunnel: w5858 -> [_ w5891]
                          frame False {
                            n3214 = local read "CAL LAB02"() -> (w5890:T16)
                          }
                          frame True {
                          }
                        }
                        n3215 = local read "LAB02 TEMP"() -> (w5866:T13)
                        n3216 = local read "TEMP LA02"() -> (w5865:T10)
                        n3217 = call "sub vi - temperature delay v4.vi"("2-run"=w5847, "1-run"=w5848, "temp values IN"=w5865, "temp signals"=w5866) -> ("T2-N"=w5860:dbl, "T2-L"=w5861:dbl, "T1-N"=w5862:dbl, "T1-L"=w5863:dbl, "temp values OUT"=w5864:T47)  [unwired: 3 in]
                        n3218 = Unbundle By Name(w5875) -> ("1 (TL) cal"=w5870:dbl, "1 (TN) cal"=w5869:dbl, "2 (TL) cal"=w5868:dbl, "2 (TN) cal"=w5867:dbl)  [unwired: 6 out]
                        n3219 = local write "TEMP LA02"(w5864) -> ()
                        n3220 = Multiply(x=w5863, y=w5870) -> (x*y=w5856:dbl)
                        n3221 = Multiply(x=w5862, y=w5869) -> (x*y=w5855:dbl)
                        n3222 = Multiply(x=w5861, y=w5868) -> (x*y=w5852:dbl)
                        n3223 = Multiply(x=w5860, y=w5867) -> (x*y=w5851:dbl)
                        n3224 = case shown="True" w5848 {
                          tunnel: w5856 -> [w5884 w5889]
                          tunnel: w5857 -> [_ w5887]
                          tunnel: [w5884 w5888] -> w5854
                          tunnel: w5855 -> [w5883 w5886]
                          tunnel: [w5883 w5885] -> w5853
                          frame False {
                          }
                          frame True {
                            n3225 = Multiply(x=w5887, y=w5886) -> (x*y=w5885:dbl)
                            n3226 = Multiply(x=w5887, y=w5889) -> (x*y=w5888:dbl)
                          }
                        }
                        n3227 = case shown="True" w5847 {
                          tunnel: w5852 -> [w5877 w5882]
                          tunnel: w5857 -> [_ w5880]
                          tunnel: [w5877 w5881] -> w5850
                          tunnel: w5851 -> [w5876 w5879]
                          tunnel: [w5876 w5878] -> w5849
                          frame False {
                          }
                          frame True {
                            n3228 = Multiply(x=w5880, y=w5879) -> (x*y=w5878:dbl)
                            n3229 = Multiply(x=w5880, y=w5882) -> (x*y=w5881:dbl)
                          }
                        }
                        n3230 = local read "SIG LAB02-2"() -> (w5872:T2)
                        n3231 = local read "SIG LAB02-1"() -> (w5874:T2)
                        n3232 = Bundle By Name(cluster=w5872, "Tmp Live"=w5850, "Tmp Neut"=w5849) -> (w5871:T2)
                        n3233 = Bundle By Name(cluster=w5874, "Tmp Live"=w5854, "Tmp Neut"=w5853) -> (w5873:T2)
                        n3234 = local write "SIG LAB02-1"(w5873) -> ()
                        n3235 = local write "SIG LAB02-2"(w5871) -> ()
                      }
                      frame #3 {
                        n3236 = case shown="False" w5904 {
                          tunnel: [w5935 w5936] -> w5920
                          tunnel: w5903 -> [_ w5936]
                          frame False {
                            n3237 = local read "CAL LAB03"() -> (w5935:T15)
                          }
                          frame True {
                          }
                        }
                        n3238 = local read "TEMP LA03"() -> (w5910:T10)
                        n3239 = local read "LAB03 TEMP"() -> (w5911:T13)
                        n3240 = call "sub vi - temperature delay v4.vi"("2-run"=w5892, "1-run"=w5893, "temp values IN"=w5910, "temp signals"=w5911) -> ("T2-N"=w5905:dbl, "T2-L"=w5906:dbl, "T1-N"=w5907:dbl, "T1-L"=w5908:dbl, "temp values OUT"=w5909:T47)  [unwired: 3 in]
